vi "Remote Antenna is Alive.vi"() -> (2 "http code":i32, 3 "alive?":bool)   [LabVIEW 2019]
panel:
  out "reply":string
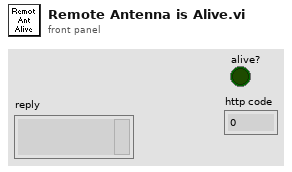
[diagram p1: front panel]
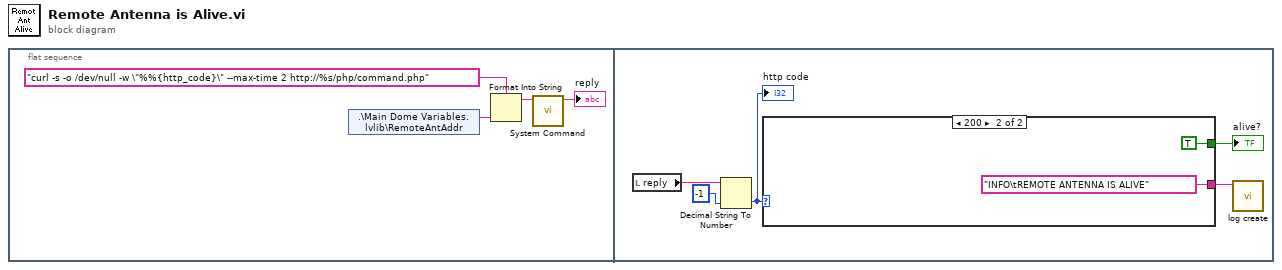
[diagram p0: block diagram]
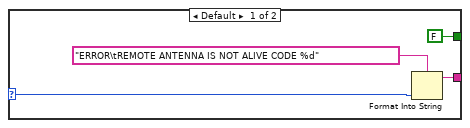
[diagram p2: hidden frame]
diagram:
  n1 = flat-sequence {
    frame #0 {
      n2 = shared-variable ".\\Main Dome Variables.lvlib\\RemoteAntAddr"() -> (w4:string)  [unwired: 1 in, 1 out]
      n3 = Format Into String(format string="curl -s -o /dev/null -w \"%%{http_code}\" --max-time 2 http://%s/php/command.php", w4) -> (resulting string=w2:string)  [unwired: 2 in, 1 out]
      n4 = call "System Command.vi"("command"=w2) -> ("standard output"=→"reply":string)  [unwired: 7 in, 3 out]
    }
    frame #1 {
      n5 = local read "reply"() -> (w8:string)
      n6 = Decimal String To Number(string=w8, default (0L)=-1 ("default (0 I32)")) -> (number=w6:i32)  [unwired: 1 in, 1 out]
      "http code" <- w6
      n7 = case shown="200" w6 {
        selector: w6 -> [w11 _]
        tunnel: [FALSE ("its ok?") TRUE ("its ok?")] -> w7
        tunnel: [w10 "INFO\tREMOTE ANTENNA IS ALIVE" ("message")] -> w5
        frame Default {
          n8 = Format Into String(format string="ERROR\tREMOTE ANTENNA IS NOT ALIVE CODE %d" ("message"), w11) -> (resulting string=w10:string)  [unwired: 2 in, 1 out]
        }
        frame 200 {
        }
      }
      "alive?" <- w7
      n9 = call "log create.vi"("message"=w5) -> ()  [unwired: 11 in]
    }
  }
